vi "Demodulacja_SSBSC.vi"(6 "Czas":dbl, 8 "Parametry_sygnalu_nosnego":T1, 9 "Czestotliwosc_probkowania":dbl, 10 "Pasmo_przenoszenia":cluster{"f_L":dbl, "f_H":dbl}, 11 "Sygnal_zmodulowany":dbl[](array[numeric])) -> (3 "Sygnal_zdemodulowany":dbl[](array[numeric]))   [LabVIEW 2020]
doc: "VI demoduluje sygnal zmodulowany metoda SSBSC"
uses:
  Kontrolki/Parametry_cosinusa.ctl
  <vilib>/Analysis/3filter.llb/Filter Passband Type.ctl
  <vilib>/Analysis/3filter.llb/Butterworth Filter (DBL).vi
  <vilib>/Analysis/NI_AALBase.lvlib
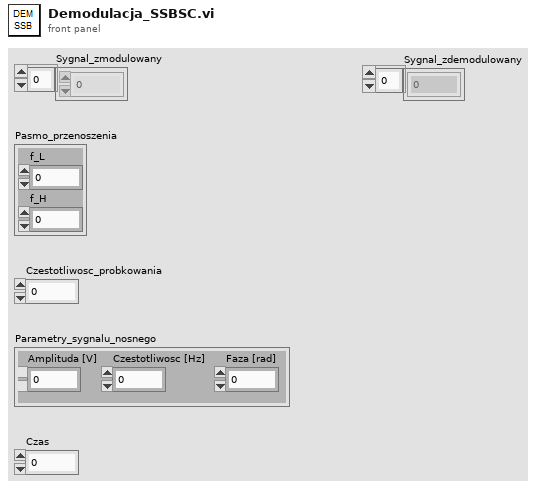
[diagram p1: front panel]
types:
  T1 = typedef "Parametry_cosinusa.ctl" = cluster{"Amplituda [V]":dbl, "Czestotliwosc [Hz] ":dbl, "Faza [rad]":dbl}
  T2 = typedef "NI_AALBase.lvlib/Filter Passband Type.ctl" = enum32{"Lowpass", "Highpass", "Bandpass", "Bandstop"}
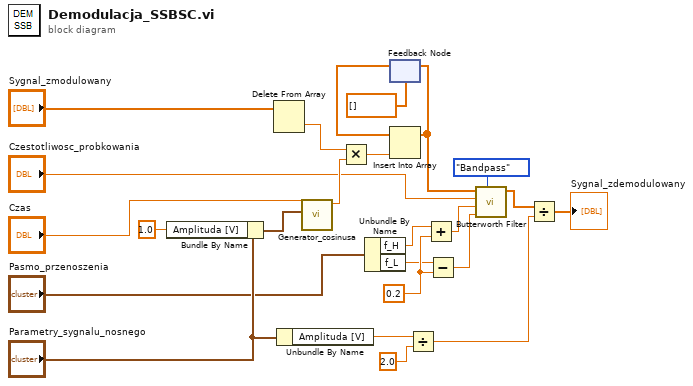
[diagram p0: block diagram]
diagram:
  w16 = 0.2
  n1 = Bundle By Name(cluster="Parametry_sygnalu_nosnego", "Amplituda [V]"=1.0) -> (w5:T1)
  n2 = Delete From Array(array="Sygnal_zmodulowany") -> (deleted portion=w4:dbl)  [unwired: 2 in, 1 out]
  n3 = Unbundle By Name("Parametry_sygnalu_nosnego") -> ("Amplituda [V]"=w20:dbl)
  n4 = call "Generator_cosinusa.vi"("Parametry_cosinusa"=w5, "Czas"="Czas") -> ("A cos(2pift + phi)"=w7:dbl)  [unwired: 9 in]
  n5 = Multiply(x=w4, y=w7) -> (x*y=w8:dbl)
  n6 = Unbundle By Name("Pasmo_przenoszenia") -> ("f_H"=w14:dbl, "f_L"=w15:dbl)
  n7 = feedback #1(dbl[] []) -> (w10:dbl[])
  n8 = Insert Into Array(array=w10, new element=w8) -> (w11:dbl[])  [unwired: 1 in]
  n9 = feedback-in #1(w11) -> ()
  n10 = Divide(x=w20, y=2.0) -> (x/y=w23:dbl)
  n11 = Add(x=w14, y=w16) -> (x+y=w17:dbl)
  n12 = Subtract(x=w15, y=w16) -> (x-y=w18:dbl)
  n13 = call-poly <vilib>:"Butterworth Filter.vi"("filter type"=Filter_Passband_Type."Bandpass", "low cutoff freq: fl"=w18, "high cutoff freq: fh"=w17, "sampling freq: fs"="Czestotliwosc_probkowania", "X"=w11) -> ("Filtered X"=w22:dbl[])  [unwired: 3 in, 1 out]
  n14 = Divide(x=w22, y=w23) -> (x/y=→"Sygnal_zdemodulowany":dbl[])
